vi "GetText.vi"(8 "error in":errorcluster, 11 "node in":refnum<class "CI Project.lvclass">) -> (0 "error out":errorcluster, 1 "additional text":string, 2 "text":string, 3 "node out":refnum<class "CI Project.lvclass">, 4 "glyph":string)   [LabVIEW 2014, in "CI Project.lvclass"]
doc: "Returns the text representation of the node used for the tree control."
uses:
  CI Project.lvclass
  CI Project.lvclass/CI Project.ctl
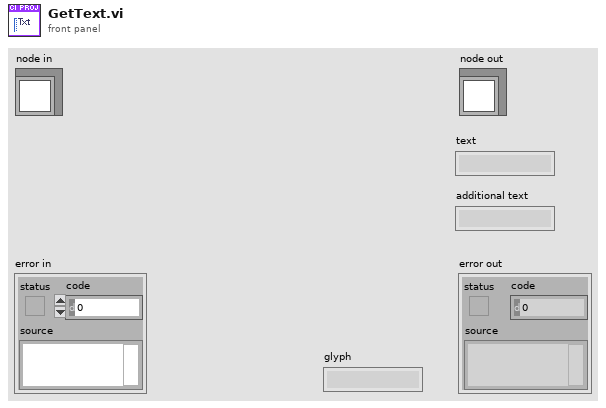
[diagram p1: front panel]
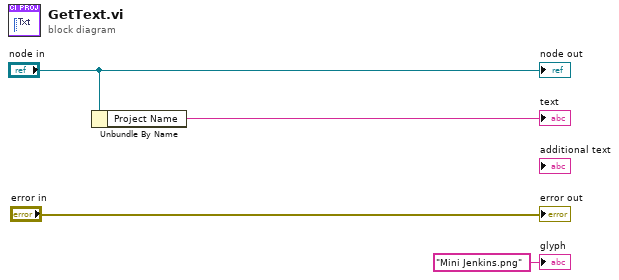
[diagram p0: block diagram]
diagram:
  n1 = Unbundle By Name("node in") -> ("Project Name"=→"text":string)
  "error out" <- "error in"
  "node out" <- "node in"
  "glyph" <- "Mini Jenkins.png" ("glyph")
